vi "Scale array2.vi"(3 "ScaleY":u8=4, 4 "ScaleX":u8=1, 5 "in Array":bool[][](array[boolean])=[[TRUE, TRUE, FALSE, TRUE, FALSE, FALSE, TRUE, FALSE, FALSE, FALSE, FALSE, TRUE, TRUE, TRUE, TRUE, FALSE, TRUE, FALSE, TRUE, TRUE, TRUE, FALSE, TRUE, TRUE, TRUE, FALSE, TRUE, TRUE, FALSE, FALSE, FALSE, TRUE, FALSE, TRUE, TRUE, TRUE, FALSE, TRUE, TRUE, FALSE, TRUE, FALSE, FALSE, FALSE, TRUE, FALSE, TRUE, TRUE, TRUE, FALSE, TRUE, TRUE, TRUE, TRUE, FALSE, TRUE, TRUE, FALSE, FALSE, TRUE, FALSE, FALSE, TRUE, TRUE, TRUE, FALSE, TRUE, TRUE, FALSE, FALSE, TRUE, TRUE, TRUE, FALSE, FALSE, TRUE, FALSE, TRUE, TRUE, FALSE, FALSE, TRUE, TRUE, FALSE, TRUE, TRUE, FALSE, FALSE, TRUE, FALSE, FALSE, FALSE, FALSE, TRUE, TRUE, FALSE, FALSE, TRUE, FALSE, TRUE, TRUE, FALSE, FALSE, FALSE, TRUE, TRUE, TRUE, FALSE, TRUE, FALSE, TRUE, TRUE]]) -> (0 "out Array":bool[][](array[boolean]))   [LabVIEW 2018]
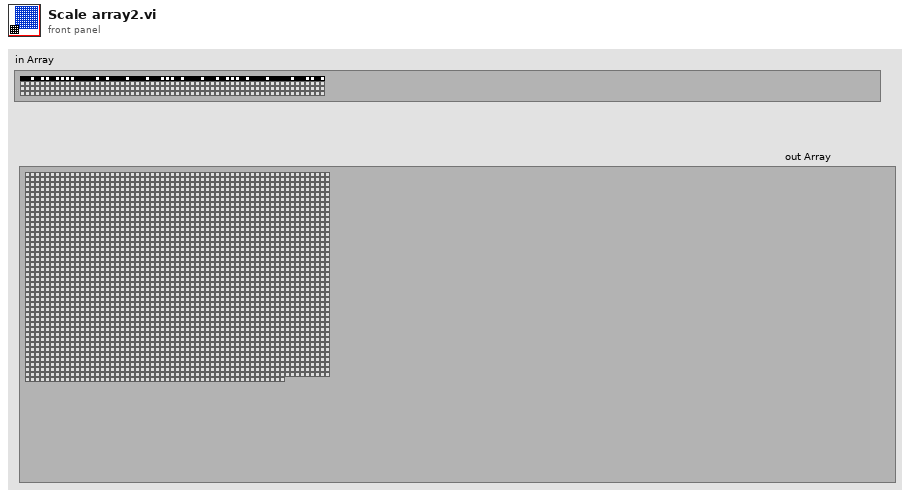
[diagram p1: front panel]
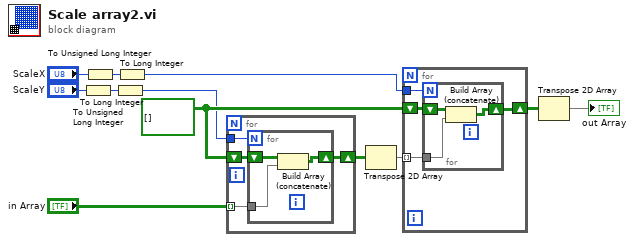
[diagram p0: block diagram]
diagram:
  w11 = bool[][] [] ("out Array")
  n1 = To Unsigned Long Integer(number="ScaleY") -> (unsigned 32bit integer=w7:u32)
  n2 = To Unsigned Long Integer(number="ScaleX") -> (unsigned 32bit integer=w4:u32)
  n3 = To Long Integer(number=w7) -> (32bit integer=w6:i32)
  n4 = To Long Integer(number=w4) -> (32bit integer=w3:i32)
  n5 = for {
    tunnel: "in Array" -> [w14] mode=indexing
    shift-right: [w13] -> w10
    shift-left: w11 -> [w16]
    tunnel: w6 -> [w15]
    n6 = for {
      N: w15 -> [_]
      tunnel: w14 -> [w17]
      shift-right: [w18] -> w13
      shift-left: w16 -> [w19]
      n7 = Build Array (concatenate)(w19, w17) -> (w18:bool[][])
    }
  }
  n8 = Transpose 2D Array(2D array=w10) -> (transposed array=w9:bool[][])
  n9 = for {
    tunnel: w9 -> [w23] mode=indexing
    tunnel: w3 -> [w22]
    shift-right: [w20] -> w8
    shift-left: w11 -> [w21]
    n10 = for {
      N: w22 -> [_]
      tunnel: w23 -> [w25]
      shift-right: [w24] -> w20
      shift-left: w21 -> [w26]
      n11 = Build Array (concatenate)(w26, w25) -> (w24:bool[][])
    }
  }
  n12 = Transpose 2D Array(2D array=w8) -> (transposed array=→"out Array":bool[][])
